vi "Launch.vi"(8 "error in (no error)":errorcluster, 10 "Run":bool, 11 "Project Instr in":refnum<class "Project Instr.lvclass">) -> (0 "error out":errorcluster, 3 "Project Instr out":refnum<class "Project Instr.lvclass">)   [LabVIEW 2015, in "Item Actor.lvlib" / "Project Instr.lvclass"]
uses:
  Project Instr.lvclass
  Instrument Information/Instrument.lvclass/Instrument.ctl
  Instrument Information/Read App Path.vi
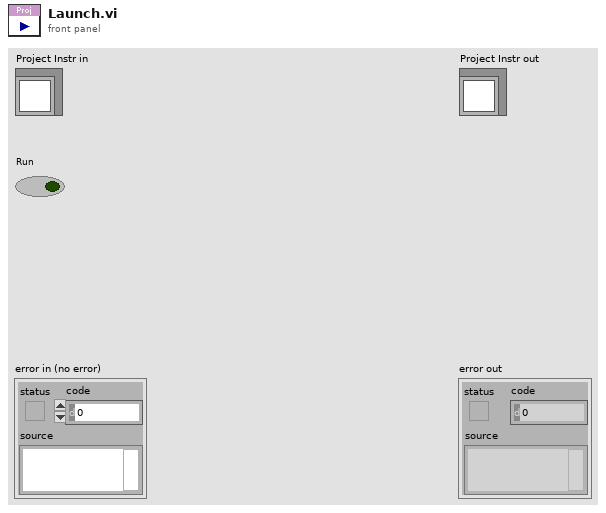
[diagram p1: front panel]
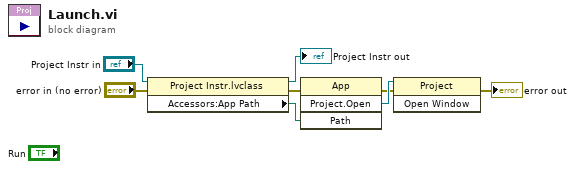
[diagram p0: block diagram]
diagram:
  n1 = property class="Project Instr.lvclass"(reference="Project Instr in", error in="error in (no error)") -> (reference out=→"Project Instr out":refnum<class "Project Instr.lvclass">, error out=w6:errorcluster, "Accessors:App Path"=w7:path)
  n2 = invoke class="App" method="Project.Open"(error in=w6, "Path"=w7) -> (error out=w1:errorcluster, "Project:Open"=w3:refnum<vi>)  [unwired: 2 in, 2 out]
  n3 = invoke class="Project" method="Open Window"(reference=w3, error in=w1) -> (error out=→"error out":errorcluster)  [unwired: 1 in, 2 out]
